vi "_PC_RTLoop_HighVolt.vi"(7 "Function":enum16{"Init", "Get Data", "Close"}(ring)=enum."Get Data", 8 "error in (no error)":errorcluster, 11 "Voltage":refnum<vi>) -> (0 "error out":errorcluster)   [LabVIEW 2018]
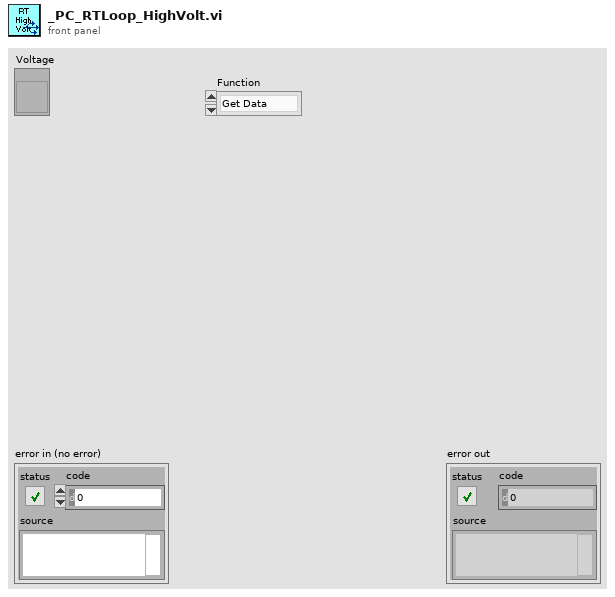
[diagram p1: front panel]
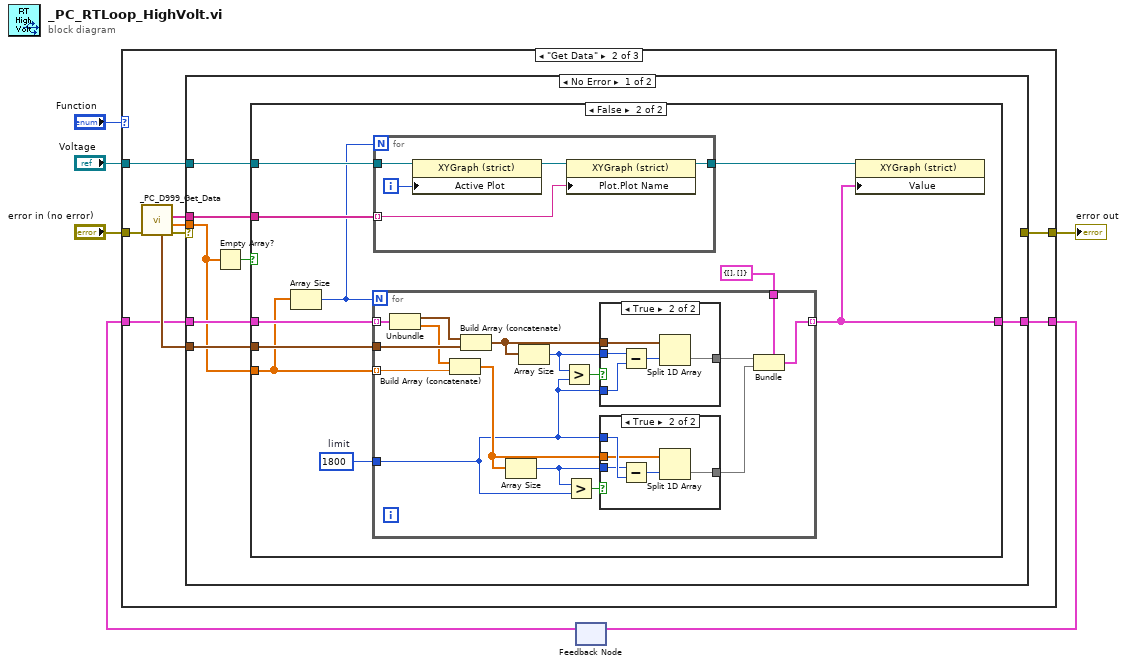
[diagram p0: block diagram]
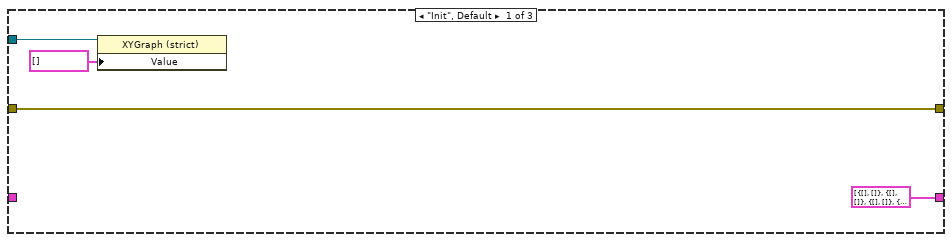
[diagram p2: hidden frame]
diagram:
  n1 = feedback #1() -> (w3:cluster{timestamp[], dbl[]}[])  [unwired: 1 in]
  n2 = case shown="\"Get Data\"" "Function" {
    tunnel: "Voltage" -> [w7 w19 _]
    tunnel: "error in (no error)" -> [w10 w14 w73]
    tunnel: [w10 w13 w73] -> w4
    tunnel: [cluster{timestamp[], dbl[]}[] [{[], []}, {[], []}, {[], []}, {[], []}, {[], []}, {[], []}, {[], []}, {[], []}, {[], []}, {[], []}, {[], []}, {[], []}] w12 _] -> w2
    tunnel: w3 -> [_ w11 _]
    frame "Init", Default {
      n3 = property class="XYGraph (strict)"(reference=w7, "Value"=cluster{timestamp[], dbl[]}[] []) -> ()  [unwired: 1 in, 2 out]
    }
    frame "Get Data" {
      n4 = call "_PC_D999_Get_Data.vi"("error in (no error)"=w14) -> ("error IO"=w15:errorcluster, "Value Array"=w16:dbl[], "Label array"=w17:string[], "timestamp"=w18:timestamp)  [unwired: 5 in, 2 out]
      n5 = case shown="No Error" w15 {
        selector: w15 -> [_ w71]
        tunnel: w18 -> [w26 _]
        tunnel: w11 -> [w25 w72]
        tunnel: w19 -> [w24 _]
        tunnel: w17 -> [w23 _]
        tunnel: [w22 w72] -> w12
        tunnel: w16 -> [w21 _]
        tunnel: [_ w71] -> w13
        frame No Error {
          n6 = Empty Array?(array=w21) -> (empty?=w20:bool)
          n7 = case shown="False" w20 {
            tunnel: w26 -> [_ w37]
            tunnel: w25 -> [w27 w36]
            tunnel: w24 -> [_ w35]
            tunnel: w23 -> [_ w33]
            tunnel: [w27 w30] -> w22
            tunnel: w21 -> [_ w31]
            frame True {
            }
            frame False {
              w29 = 1800  # limit
              n8 = Array Size(array=w31) -> (size(s)=w32:i32)
              n9 = for {
                N: w32 -> [_]
                tunnel: w31 -> [w54] mode=indexing
                tunnel: w37 -> [w56]
                tunnel: w36 -> [w58] mode=indexing
                tunnel: [w52] -> w30 mode=indexing
                tunnel: cluster{timestamp[], dbl[]} {[], []} -> [w53]
                tunnel: w29 -> [w45]
                n10 = Unbundle(w58) -> (w57:timestamp[], w55:dbl[])
                n11 = Build Array (concatenate)(w55, w54) -> (w46:dbl[])
                n12 = Build Array (concatenate)(w57, w56) -> (w51:timestamp[])
                n13 = Array Size(array=w46) -> (size(s)=w48:i32)
                n14 = Array Size(array=w51) -> (size(s)=w50:i32)
                n15 = Greater?(x=w50, y=w45) -> (0:w49:bool)
                n16 = Greater?(x=w48, y=w45) -> (0:w47:bool)
                n17 = case shown="True" w49 {
                  tunnel: w45 -> [_ w70]
                  tunnel: w50 -> [_ w69]
                  tunnel: [w65 w67] -> w44
                  tunnel: w51 -> [w65 w66]
                  frame False {
                  }
                  frame True {
                    n18 = Subtract(x=w69, y=w70) -> (x-y=w68:i32)
                    n19 = Split 1D Array(array=w66, index=w68) -> (second subarray=w67:timestamp[])  [unwired: 1 out]
                  }
                }
                n20 = case shown="True" w47 {
                  tunnel: w45 -> [_ w64]
                  tunnel: w48 -> [_ w63]
                  tunnel: [w59 w61] -> w43
                  tunnel: w46 -> [w59 w60]
                  frame False {
                  }
                  frame True {
                    n21 = Subtract(x=w63, y=w64) -> (x-y=w62:i32)
                    n22 = Split 1D Array(array=w60, index=w62) -> (second subarray=w61:dbl[])  [unwired: 1 out]
                  }
                }
                n23 = Bundle(cluster=w53, w44, w43) -> (w52:cluster{timestamp[], dbl[]})
              }
              n24 = for {
                N: w32 -> [_]
                tunnel: w35 -> [w42]
                tunnel: [w40] -> w34
                tunnel: w33 -> [w39] mode=indexing
                i -> [w38]
                n25 = property class="XYGraph (strict)"(reference=w42, "Active Plot"=w38) -> (reference out=w41:refnum<vi>)  [unwired: 1 in, 1 out]
                n26 = property class="XYGraph (strict)"(reference=w41, "Plot.Plot Name"=w39) -> (reference out=w40:refnum<vi>)  [unwired: 1 in, 1 out]
              }
              n27 = property class="XYGraph (strict)"(reference=w34, "Value"=w30) -> ()  [unwired: 1 in, 2 out]
            }
          }
        }
        frame Error {
        }
      }
    }
    frame "Close" {
    }
  }
  "error out" <- w4
  n28 = feedback-in #1(w2) -> ()
